vi "Engine Out - Faults - Engine Speed.vi"(11 "Engine Speed [RPM]":sgl) -> ()   [LabVIEW 2015, in "ECS-RT.lvlib"]
uses:
  ECS-RT.lvlib
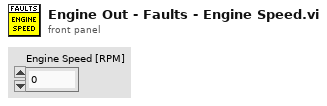
[diagram p1: front panel]
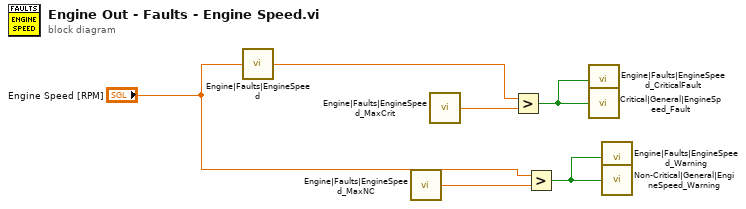
[diagram p0: block diagram]
diagram:
  n1 = call "Engine|Faults|EngineSpeed"("Value"="Engine Speed [RPM]") -> ()
  n2 = call "Engine|Faults|EngineSpeed_MaxNC"() -> ("Value"=w4:sgl)
  n3 = call "Engine|Faults|EngineSpeed_MaxCrit"() -> ("Value"=w2:sgl)
  n4 = Greater?(x="Engine Speed [RPM]", y=w2) -> (0:w3:bool)
  n5 = Greater?(x="Engine Speed [RPM]", y=w4) -> (0:w5:bool)
  n6 = call "Engine|Faults|EngineSpeed_CriticalFault"("Value"=w3) -> ()
  n7 = call "Critical|General|EngineSpeed_Fault"("Fault"=w3) -> ()  [unwired: 2 in]
  n8 = call "Engine|Faults|EngineSpeed_Warning"("Value"=w5) -> ()
  n9 = call "Non-Critical|General|EngineSpeed_Warning"("Fault"=w5) -> ()  [unwired: 2 in]
